vi "获取剖面数据.vi"(8 "end time":timestamp, 9 "start time":timestamp, 10 "测量模式":string="水样测试", 11 "table":string="剖面多参数") -> (1 "数组":T1(array[cluster]) {"污染物" items=["水温"=1, "浊度"=2, "DO"=3, "pH"=4, "ORP"=5, "比电导率"=6, "叶绿素a"=7, "氨氮"=8, "亚硝氮"=9, "硫化物"=10, "电压"=11, "温度"=12, "湿度"=13, "GPS经度"=14, "GPS纬度"=15, "BD经度"=16, "BD纬度"=17]; "标识" items=["N"=1, "T"=2, "L"=3, "D"=4, "Z"=5, "M"=6, "hd"=7]}, 2 "有数据":bool, 3 "table 2":string)   [LabVIEW 2016, in "环境动力监测库.lvlib" / "NMEA.lvlib"]
uses:
  NMEA.lvlib
  <vilib>/addons/database/_DB Variant To Data/Database Variant To Data.xnode
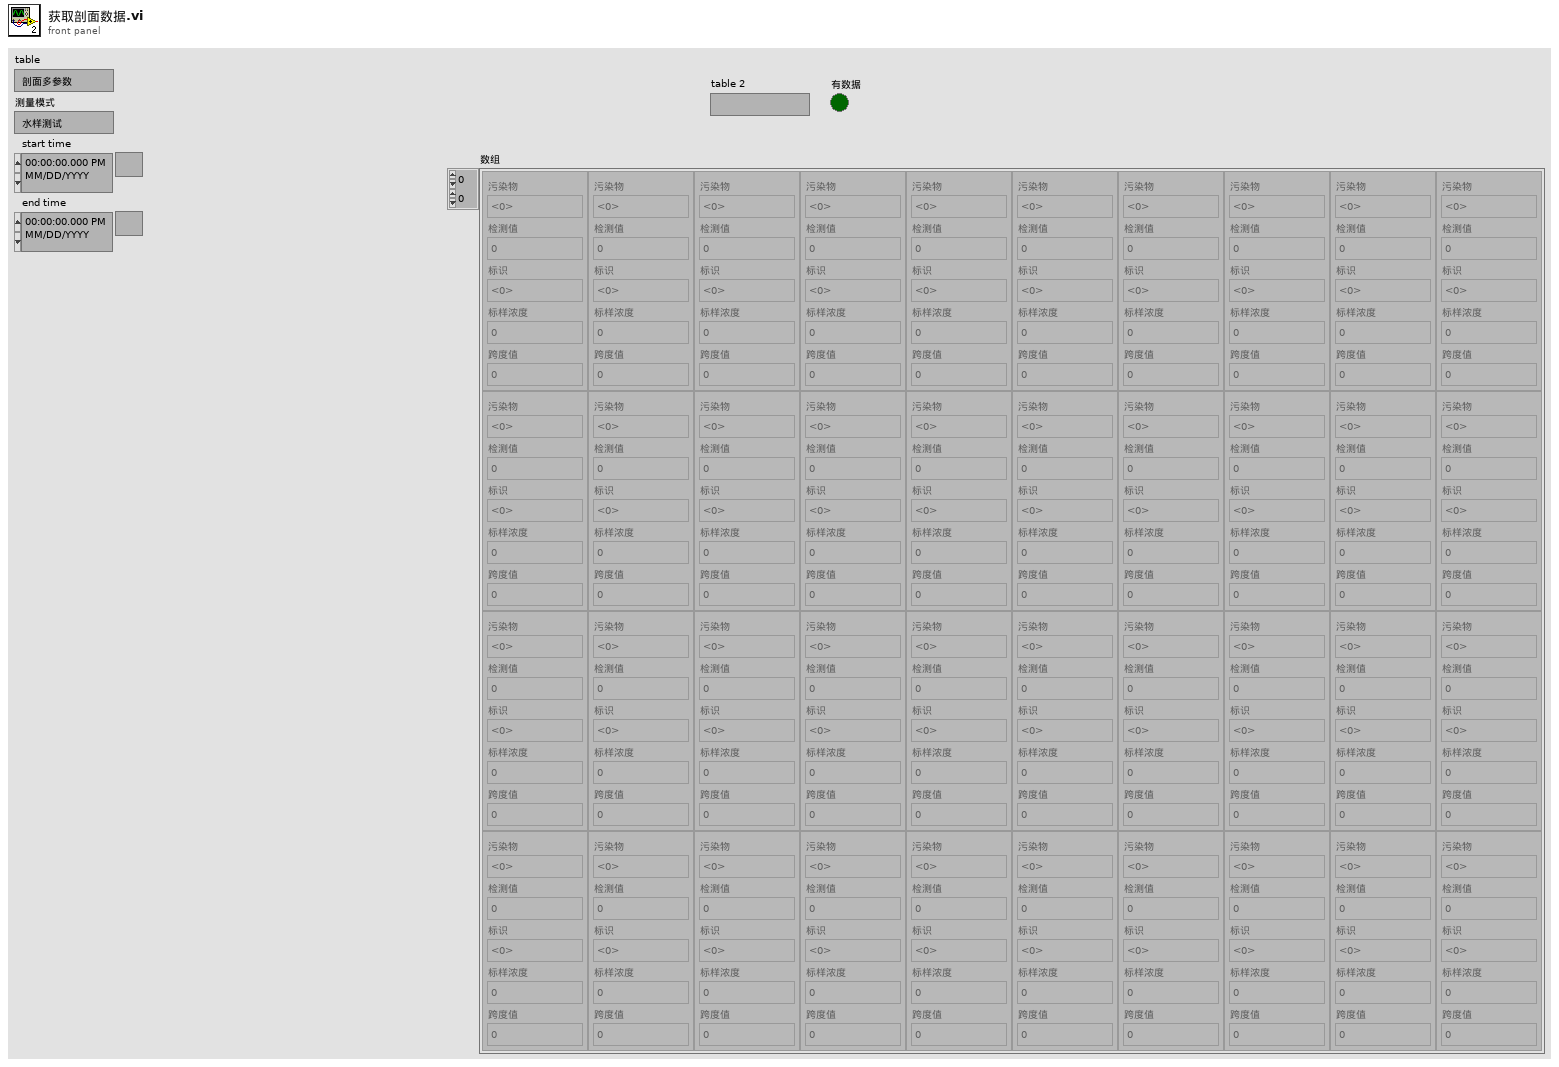
[diagram p1: front panel]
types:
  T1 = cluster{"污染物":u16, "检测值":dbl, "标识":u16, "标样浓度":dbl, "跨度值":dbl}[][]
  T2 = cluster{"时间标识":timestamp, "测量模式":string, "数据标识":string, "层数":u16, "temp":dbl, "Spcond":dbl, "pH":dbl, "ORP":dbl, "ODO":dbl, "Turb":dbl, "Chla":dbl}[]
  T3 = cluster{"污染物":u16, "检测值":dbl, "标识":u16, "标样浓度":dbl, "跨度值":dbl}[]
  T4 = cluster{"污染物":u16, "检测值":dbl, "标识":u16, "标样浓度":dbl, "跨度值":dbl}
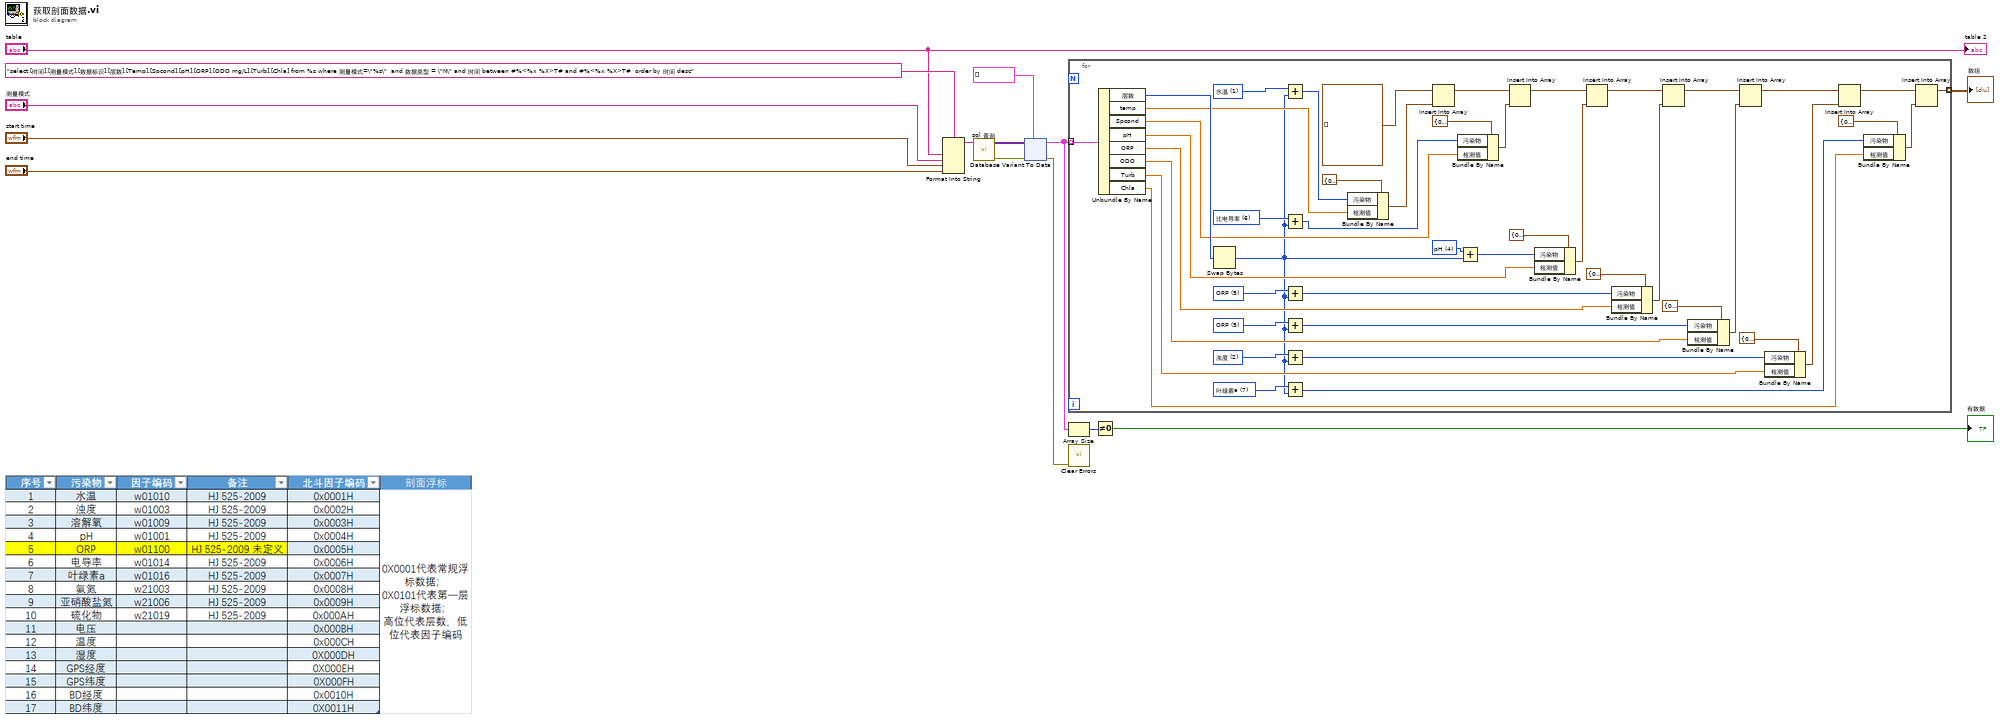
[diagram p0: block diagram]
diagram:
  n1 = Format Into String(format string="select [时间],[测量模式],[数据标识],[层数],[Temp],[Spcond],[pH],[ORP],[ODO mg/L],[Turb],[Chla] from %s where 测量模式=\"%s\"  and 数据类型 = \"N\" and 时间 between #%<%x %X>T# and #%<%x %X>T#  order by 时间 desc" ("格式字符串"), "table", "测量模式", "start time", "end time") -> (resulting string=w12:string)  [unwired: 2 in, 1 out]
  n2 = call "sql 查询.vi"("SQL query"=w12) -> ("error out"=w9:errorcluster, "recordset data"=w11:variant[][])  [unwired: 9 in]
  n3 = xnode "Database Variant To Data"("database variant"=w11, "error in (no error)"=w9, "type"=T2 []) -> ("data"=w3:T2, "error out"=w1:errorcluster)
  n4 = for {
    tunnel: w3 -> [w60] mode=indexing
    tunnel: [w16] -> w2 mode=indexing
    w21 = u16 7 items=["水温"=1, "浊度"=2, "DO"=3, "pH"=4, "ORP"=5, "比电导率"=6, "叶绿素a"=7, "氨氮"=8, "亚硝氮"=9, "硫化物"=10, "电压"=11, "温度"=12, "湿度"=13, "GPS经度"=14, "GPS纬度"=15, "BD经度"=16, "BD纬度"=17] ("污染物")
    w28 = u16 2 items=["水温"=1, "浊度"=2, "DO"=3, "pH"=4, "ORP"=5, "比电导率"=6, "叶绿素a"=7, "氨氮"=8, "亚硝氮"=9, "硫化物"=10, "电压"=11, "温度"=12, "湿度"=13, "GPS经度"=14, "GPS纬度"=15, "BD经度"=16, "BD纬度"=17] ("污染物")
    w33 = u16 5 items=["水温"=1, "浊度"=2, "DO"=3, "pH"=4, "ORP"=5, "比电导率"=6, "叶绿素a"=7, "氨氮"=8, "亚硝氮"=9, "硫化物"=10, "电压"=11, "温度"=12, "湿度"=13, "GPS经度"=14, "GPS纬度"=15, "BD经度"=16, "BD纬度"=17] ("污染物")
    w40 = u16 5 items=["水温"=1, "浊度"=2, "DO"=3, "pH"=4, "ORP"=5, "比电导率"=6, "叶绿素a"=7, "氨氮"=8, "亚硝氮"=9, "硫化物"=10, "电压"=11, "温度"=12, "湿度"=13, "GPS经度"=14, "GPS纬度"=15, "BD经度"=16, "BD纬度"=17] ("污染物")
    w45 = u16 4 items=["水温"=1, "浊度"=2, "DO"=3, "pH"=4, "ORP"=5, "比电导率"=6, "叶绿素a"=7, "氨氮"=8, "亚硝氮"=9, "硫化物"=10, "电压"=11, "温度"=12, "湿度"=13, "GPS经度"=14, "GPS纬度"=15, "BD经度"=16, "BD纬度"=17] ("污染物")
    w52 = u16 6 items=["水温"=1, "浊度"=2, "DO"=3, "pH"=4, "ORP"=5, "比电导率"=6, "叶绿素a"=7, "氨氮"=8, "亚硝氮"=9, "硫化物"=10, "电压"=11, "温度"=12, "湿度"=13, "GPS经度"=14, "GPS纬度"=15, "BD经度"=16, "BD纬度"=17] ("污染物")
    w56 = u16 1 items=["水温"=1, "浊度"=2, "DO"=3, "pH"=4, "ORP"=5, "比电导率"=6, "叶绿素a"=7, "氨氮"=8, "亚硝氮"=9, "硫化物"=10, "电压"=11, "温度"=12, "湿度"=13, "GPS经度"=14, "GPS纬度"=15, "BD经度"=16, "BD纬度"=17] ("污染物")
    n5 = Unbundle By Name(w60) -> ("层数"=w57:u16, "temp"=w54:dbl, "Spcond"=w48:dbl, "pH"=w42:dbl, "ORP"=w36:dbl, "ODO"=w30:dbl, "Turb"=w24:dbl, "Chla"=w18:dbl)
    n6 = Swap Bytes(anything=w57) -> (byte swapped=w15:u16)
    n7 = Add(x=w56, y=w15) -> (x+y=w55:u16)
    n8 = Add(x=w52, y=w15) -> (x+y=w53:u16)
    n9 = Add(x=w40, y=w15) -> (x+y=w41:u16)
    n10 = Add(x=w33, y=w15) -> (x+y=w32:u16)
    n11 = Add(x=w28, y=w15) -> (x+y=w29:u16)
    n12 = Add(x=w21, y=w15) -> (x+y=w20:u16)
    n13 = Bundle By Name(cluster=T4 {"污染物"=0, "检测值"=0.0, "标识"=1, "标样浓度"=0.0, "跨度值"=0.0} ("数据"), "污染物"=w55, "检测值"=w54) -> (w58:T4)
    n14 = Insert Into Array(array=T3 [] ("数组"), new element=w58) -> (w49:T3)  [unwired: 1 in]
    n15 = Bundle By Name(cluster=T4 {"污染物"=0, "检测值"=0.0, "标识"=1, "标样浓度"=0.0, "跨度值"=0.0} ("数据"), "污染物"=w53, "检测值"=w48) -> (w51:T4)
    n16 = Add(x=w45, y=w15) -> (x+y=w44:u16)
    n17 = Insert Into Array(array=w49, new element=w51) -> (w43:T3)  [unwired: 1 in]
    n18 = Bundle By Name(cluster=T4 {"污染物"=0, "检测值"=0.0, "标识"=1, "标样浓度"=0.0, "跨度值"=0.0} ("数据"), "污染物"=w44, "检测值"=w42) -> (w46:T4)
    n19 = Insert Into Array(array=w43, new element=w46) -> (w37:T3)  [unwired: 1 in]
    n20 = Bundle By Name(cluster=T4 {"污染物"=0, "检测值"=0.0, "标识"=1, "标样浓度"=0.0, "跨度值"=0.0} ("数据"), "污染物"=w41, "检测值"=w36) -> (w39:T4)
    n21 = Insert Into Array(array=w37, new element=w39) -> (w31:T3)  [unwired: 1 in]
    n22 = Bundle By Name(cluster=T4 {"污染物"=0, "检测值"=0.0, "标识"=1, "标样浓度"=0.0, "跨度值"=0.0} ("数据"), "污染物"=w32, "检测值"=w30) -> (w34:T4)
    n23 = Insert Into Array(array=w31, new element=w34) -> (w25:T3)  [unwired: 1 in]
    n24 = Bundle By Name(cluster=T4 {"污染物"=0, "检测值"=0.0, "标识"=1, "标样浓度"=0.0, "跨度值"=0.0} ("数据"), "污染物"=w29, "检测值"=w24) -> (w27:T4)
    n25 = Insert Into Array(array=w25, new element=w27) -> (w19:T3)  [unwired: 1 in]
    n26 = Bundle By Name(cluster=T4 {"污染物"=0, "检测值"=0.0, "标识"=1, "标样浓度"=0.0, "跨度值"=0.0} ("数据"), "污染物"=w20, "检测值"=w18) -> (w22:T4)
    n27 = Insert Into Array(array=w19, new element=w22) -> (w16:T3)  [unwired: 1 in]
  }
  "数组" <- w2
  n28 = Array Size(array=w3) -> (size(s)=w5:i32)
  n29 = call <vilib>:"Clear Errors.vi"("error in (no error)"=w1) -> ()  [unwired: 5 in, 2 out]
  n30 = Not Equal To 0?(x=w5) -> (x != 0?=→"有数据":bool)
  "table 2" <- "table"
